vi "FLS.vi"(0 "System no.":i32=1 min=1 step=1, 1 "Board":i32=1 min=1 max=5 step=1, 2 "Axis to scan":string, 3 "Scan direction":u16(ring)=2 items=["Scan left & right (- & +)", "Scan only left (-)", "Scan only right (+)"], 4 "Range":dbl=0.1 format="%.4f", 5 "error in":errorcluster, 6 "Treshold level":dbl=0.1 format="%.3f", 7 "Step size":dbl=0.001 format="%.4f", 8 "Decrease VEL\nfor scan?":bool, 9 "Velocity":dbl=0.2 format="%.4f", 10 "Use #7 polling?":bool=TRUE, 11 "Timeout (s)":dbl=300.0 min=1.0 max=4.0 step=1.0 format="%.2f", 12 "Stop refnum":refnum<vi>) -> (14 "Scan successful?":bool, 15 "Controller error":bool, 19 "error out":errorcluster)   [LabVIEW 2026]
doc: "Performs a line scan specified axis, waits until scan is ready (using #7 polling if checked) and indicates whether scan was successful or not. Velocity is only valid if Decrease VEL for scan? Is TRUE. If Decrease VEL for scan? is TRUE, velocity is decreased before and reset after the scan. Timeout is only valid if Use #7 polling is FALSE. If Refnum stop or Local stop is TRUE, VI sends #24 and stops. When using as a sub-VI, use Refnum stop to stop VI from caller.\n\nC-880: Use #7 polling? = TRUE\n\nC-887, F-206, M-8X0: Use #7 polling? = FALSE. Only for GCS syntax version = GCS 2.0 or higher (check with CSV?.vi. If CSV?.vi is not supported, syntax version is GCS 1.0). Step size is not valid."
uses:
  Communication/Syntax.ctl
  GeneralCommands/Controller names.ctl
  Communication/Global1.vi
  GeneralCommands/Global2 (Array).vi
panel:
  in  "Local stop":bool
  # "Performs a line scan in specified axis, waits until scan is ready (using #7 polling if \nchecked) and indicates whether scan was successful or not. If Stop refnum or \nLocal stop is TRUE, VI sends #24 and stops. \"Velocity\" is only valid if \"Decrease VEL \nfor scan?\" Is TRUE.  If \"Decrease VEL for scan?\" is TRUE, velocity is decreased before \nand reset after the scan. \"Timeout\" is only valid if \"Use #7 polling\" is FALSE."
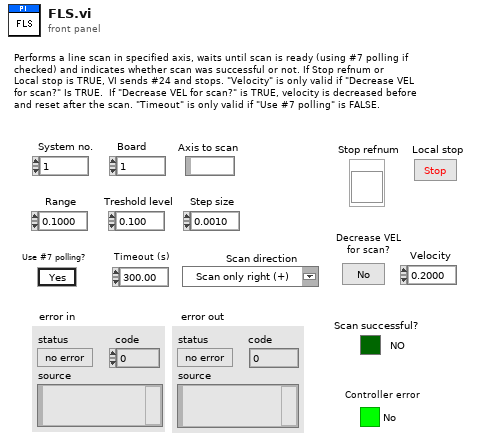
[diagram p1: front panel]
types:
  T1 = typedef "Syntax.ctl" = enum16{"GCS 1.0", "GCS 2.0", "GCS 3.0"}
  T2 = typedef "Controller names.ctl" = enum16{"None", "Analog", "C-702", "C-413", "C-414", "C-843", "C-843.PM", "C-844", "C-848", "C-865", "C-866", "C-867", "C-877", "C-880", "C-884", "C-885", "C-886", "C-887", "C-891", "E-135", "E-516", "E-517", "E-518", "E-709", "E-710", "E-712", "E-725", "E-727", "E-753", "E-754", "E-755", "E-761", "E-816", "E-861", "E-870", "E-871", "E-872", "E-873", "E-874", "F-206", "HydraPollux", "M-840", "M-850", "M-8X0", "Mercury", "Mercury_GCS", "PI_GCS2"}
  T3 = cluster{"Conn. axes":string[], "Controller name":T2}[]
  T4 = cluster{"Conn. axes":string[], "Controller name":T2}
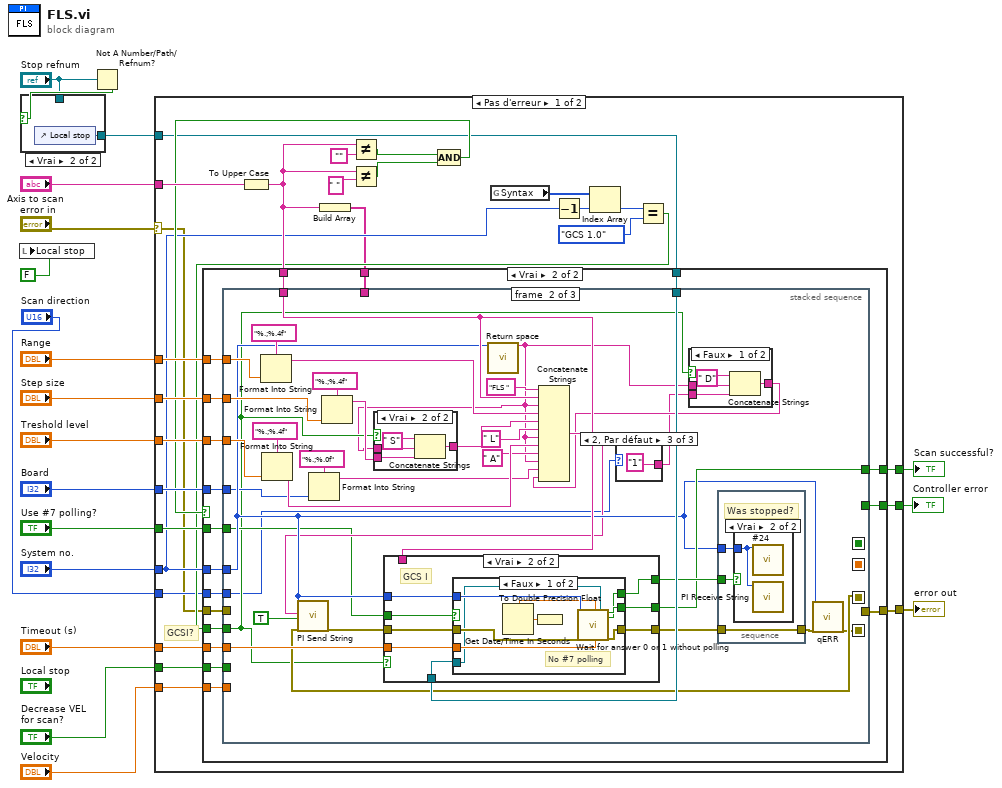
[diagram p0: block diagram]
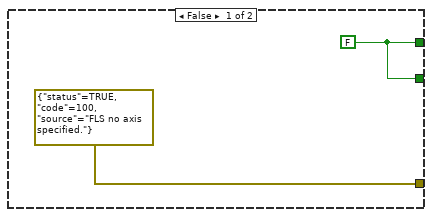
[diagram p3: hidden frame]
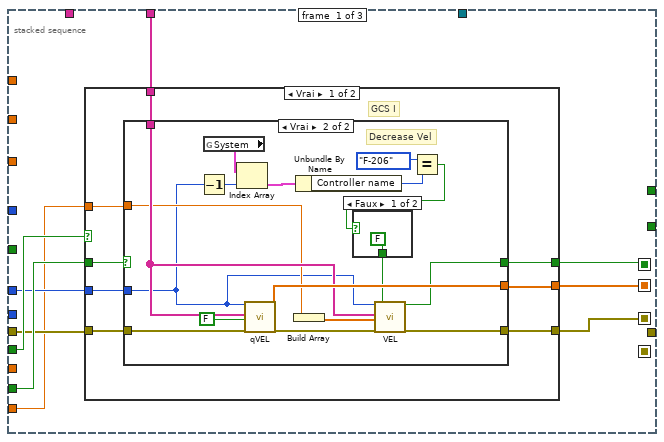
[diagram p4: hidden frame]
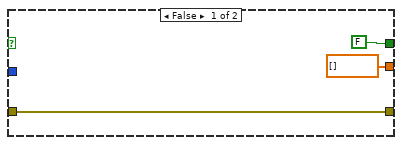
[diagram p5: hidden frame]
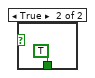
[diagram p6: hidden frame]
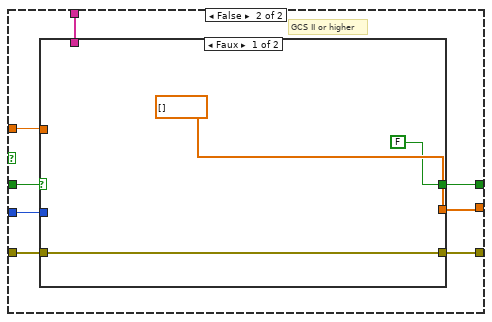
[diagram p7: hidden frame]
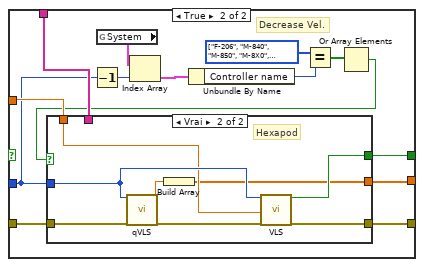
[diagram p8: hidden frame]
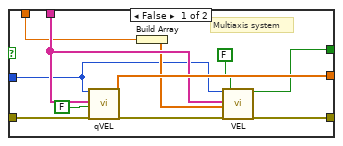
[diagram p9: hidden frame]
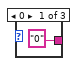
[diagram p10: hidden frame]
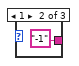
[diagram p11: hidden frame]
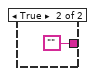
[diagram p12: hidden frame]
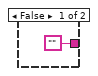
[diagram p13: hidden frame]
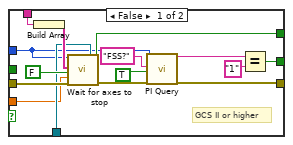
[diagram p14: hidden frame]
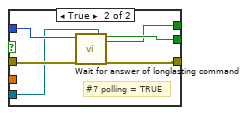
[diagram p15: hidden frame]
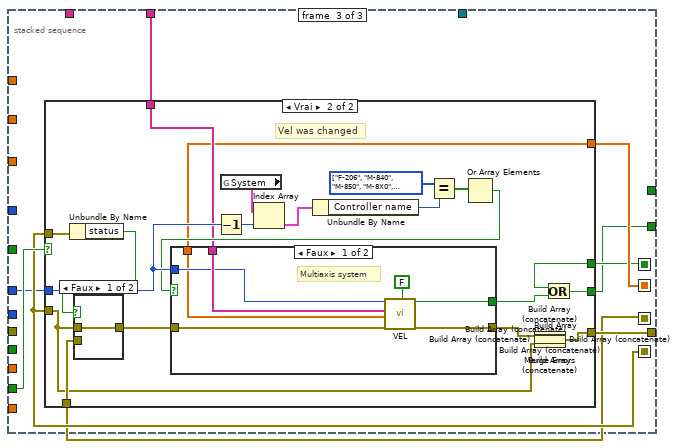
[diagram p17: hidden frame]
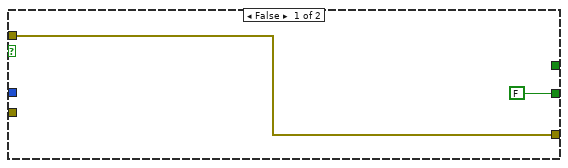
[diagram p18: hidden frame]
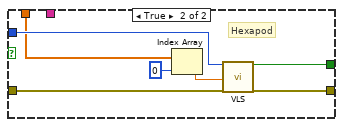
[diagram p19: hidden frame]
diagram:
  n1 = local write "Local stop"(FALSE ("Local stop")) -> ()
  n2 = Not A Number/Path/Refnum?(number/path/refnum="Stop refnum") -> (NaN/Path/Refnum?=w10:bool)
  n3 = case shown="Vrai" w10 {
    tunnel: [w20 w21] -> w8
    tunnel: "Stop refnum" -> [w20 _]
    frame False {
    }
    frame True {
      n4 = control-ref of="Local stop"() -> (w21:refnum<vi>)
    }
  }
  n5 = case shown="Pas d'erreur" "error in" {
    selector: "error in" -> [w23 w297]
    tunnel: "System no." -> [w30 _]
    tunnel: [w38 w297] -> w18
    tunnel: "Axis to scan" -> [w49 _]
    tunnel: [w37 w298] -> w16
    tunnel: "Board" -> [w44 _]
    tunnel: "Range" -> [w43 _]
    tunnel: "Step size" -> [w42 _]
    tunnel: "Treshold level" -> [w40 _]
    tunnel: w8 -> [w36 _]
    tunnel: "Use #7 polling?" -> [w35 _]
    tunnel: "Timeout (s)" -> [w34 _]
    tunnel: "Decrease VEL\nfor scan?" -> [w28 _]
    tunnel: "Velocity" -> [w27 _]
    tunnel: [w25 w298] -> w3
    tunnel: "Scan direction" -> [w24 _]
    frame No Error {
      # "GCSI?"
      n6 = To Upper Case(1:w49) -> (0:w41:string)
      n7 = Build Array(w41) -> (w26:string[])
      n8 = Not Equal?(x=w41, y="") -> (x != y?=w46:bool)
      n9 = Not Equal?(x=w41, y=" ") -> (x != y?=w45:bool)
      n10 = Compound Arithmetic op=AND(w46, w45) -> (w39:bool)
      n11 = global read "Global1.vi" "Syntax"() -> (w31:T1[])
      n12 = Decrement(x=w30) -> (x-1=w32:i32)
      n13 = Index Array(array=w31, index=w32) -> (element=w33:T1)
      n14 = Equal?(x=w33, y=Syntax."GCS 1.0") -> (x = y?=w29:bool)
      n15 = case shown="Vrai" w39 {
        tunnel: w44 -> [_ w58]
        tunnel: w43 -> [_ w68]
        tunnel: w42 -> [_ w66]
        tunnel: w41 -> [_ w63]
        tunnel: w40 -> [_ w67]
        tunnel: w23 -> [_ w69]
        tunnel: w30 -> [_ w59]
        tunnel: [errorcluster {"status"=TRUE, "code"=100, "source"="FLS no axis specified."} ("error out") w65] -> w38
        tunnel: [w50 w61] -> w37
        tunnel: w36 -> [_ w62]
        tunnel: w35 -> [_ w64]
        tunnel: w34 -> [_ w60]
        tunnel: w29 -> [_ w57]
        tunnel: w28 -> [_ w56]
        tunnel: w27 -> [_ w55]
        tunnel: w26 -> [_ w54]
        tunnel: [w50 w53] -> w25
        tunnel: w24 -> [_ w52]
        frame False {
          w50 = FALSE
        }
        frame True {
          n16 = stacked-sequence {
            seq-local: [w74 _ _] -> [_ w162 w247]
            seq-local: [w73 _ _] -> [_ _ w244]
            seq-local: [w70 _ _] -> [_ _ w245]
            seq-local: [_ w161 _] -> [_ _ w249]
            tunnel: w69 -> [w75 _ _]
            tunnel: w68 -> [_ w185 _]
            tunnel: w67 -> [_ w182 _]
            tunnel: w66 -> [_ w180 _]
            tunnel: [_ _ w250] -> w65
            tunnel: w64 -> [_ w160 _]
            tunnel: w63 -> [_ w174 _]
            tunnel: w62 -> [_ w173 _]
            tunnel: [_ w170 _] -> w61
            tunnel: w60 -> [_ w169 _]
            tunnel: w59 -> [w76 w168 w248]
            tunnel: w58 -> [_ w165 _]
            tunnel: w57 -> [w78 w156 _]
            tunnel: w56 -> [w77 _ w251]
            tunnel: w55 -> [w72 _ _]
            tunnel: w54 -> [w71 _ w246]
            tunnel: [_ _ w243] -> w53
            tunnel: w52 -> [_ w154 _]
            frame #0 {
              n17 = case shown="Vrai" w78 {
                tunnel: w71 -> [w83 w113]
                tunnel: w75 -> [w86 w116]
                tunnel: [w85 w115] -> w70
                tunnel: w76 -> [w80 w110]
                tunnel: [w84 w114] -> w74
                tunnel: w72 -> [w82 w112]
                tunnel: [w81 w111] -> w73
                tunnel: w77 -> [w79 w109]
                frame True {
                  # "GCS I"
                  n18 = case shown="Vrai" w79 {
                    tunnel: w86 -> [w87 w105]
                    tunnel: [dbl[] [] ("Velocity") w104] -> w85
                    tunnel: [w87 w102] -> w84
                    tunnel: w83 -> [_ w101]
                    tunnel: w82 -> [_ w100]
                    tunnel: [FALSE ("Controller error") w98] -> w81
                    tunnel: w80 -> [_ w96]
                    frame False {
                    }
                    frame True {
                      # "Decrease Vel"
                      n19 = Decrement(x=w96) -> (x-1=w95:i32)
                      n20 = global read "Global2 (Array).vi" "System"() -> (w97:T3)
                      n21 = Index Array(array=w97, index=w95) -> (element=w94:T4)
                      n22 = call "qVEL.vi"("System no."=w96, "Axes to query"=w101, "All axes?"=FALSE, "error in"=w105) -> ("Velocity"=w104:dbl[], "error out"=w103:errorcluster)  [unwired: 1 in, 13 out]
                      n23 = Build Array(w100) -> (w99:dbl[])
                      n24 = Unbundle By Name(w94) -> ("Controller name"=w93:T2)
                      n25 = Equal?(x=Controller_names."F-206" ("Controller name"), y=w93) -> (x = y?=w91:bool)
                      n26 = case shown="Faux" w91 {
                        tunnel: [FALSE ("Without axis ID?") TRUE ("Without axis ID?")] -> w90
                        frame False {
                        }
                        frame True {
                        }
                      }
                      n27 = call "VEL.vi"("System no."=w96, "Axes to set"=w101, "Velocity values"=w99, "error in"=w103, "Without axis ID?"=w90) -> ("Controller error"=w98:bool, "error out"=w102:errorcluster)  [unwired: 1 in, 12 out]
                    }
                  }
                }
                frame False {
                  # "GCS II or higher"
                  n28 = case shown="Faux" w109 {
                    tunnel: w116 -> [w117 w133]
                    tunnel: [dbl[] [] ("Velocity") w132] -> w115
                    tunnel: [w117 w131] -> w114
                    tunnel: w113 -> [_ w130]
                    tunnel: w112 -> [_ w129]
                    tunnel: [FALSE ("Controller error") w128] -> w111
                    tunnel: w110 -> [_ w126]
                    frame False {
                    }
                    frame True {
                      w122 = T2[] [enum."F-206", enum."M-840", enum."M-850", enum."M-8X0", enum."C-887"] items=["None", "Analog", "C-702", "C-413", "C-414", "C-843", "C-843.PM", "C-844", "C-848", "C-865", "C-866", "C-867", "C-877", "C-880", "C-884", "C-885", "C-886", "C-887", "C-891", "E-135", "E-516", "E-517", "E-518", "E-709", "E-710", "E-712", "E-725", "E-727", "E-753", "E-754", "E-755", "E-761", "E-816", "E-861", "E-870", "E-871", "E-872", "E-873", "E-874", "F-206", "HydraPollux", "M-840", "M-850", "M-8X0", "Mercury", "Mercury_GCS", "PI_GCS2"]
                      # "Decrease Vel."
                      n29 = Decrement(x=w126) -> (x-1=w125:i32)
                      n30 = global read "Global2 (Array).vi" "System"() -> (w127:T3)
                      n31 = Index Array(array=w127, index=w125) -> (element=w124:T4)
                      n32 = Unbundle By Name(w124) -> ("Controller name"=w123:T2)
                      n33 = Equal?(x=w122, y=w123) -> (x = y?=w121:bool[])
                      n34 = Or Array Elements(Boolean array=w121) -> (logical OR=w120:bool)
                      n35 = case shown="Vrai" w120 {
                        tunnel: w133 -> [w143 w152]
                        tunnel: [w142 w145] -> w132
                        tunnel: [w140 w150] -> w131
                        tunnel: w130 -> [w139 _]
                        tunnel: w129 -> [w138 w147]
                        tunnel: [w136 w149] -> w128
                        tunnel: w126 -> [w135 w148]
                        frame False {
                          # "Multiaxis system"
                          n36 = call "qVEL.vi"("System no."=w135, "Axes to query"=w139, "All axes?"=FALSE, "error in"=w143) -> ("Velocity"=w142:dbl[], "error out"=w141:errorcluster)  [unwired: 1 in, 13 out]
                          n37 = Build Array(w138) -> (w137:dbl[])
                          n38 = call "VEL.vi"("System no."=w135, "Axes to set"=w139, "Velocity values"=w137, "error in"=w141, "Without axis ID?"=FALSE) -> ("Controller error"=w136:bool, "error out"=w140:errorcluster)  [unwired: 1 in, 12 out]
                        }
                        frame True {
                          # "Hexapod"
                          n39 = call "qVLS.vi"("System no."=w148, "error in"=w152) -> ("Velocity"=w146:dbl, "error out"=w151:errorcluster)  [unwired: 2 in, 14 out]
                          n40 = Build Array(w146) -> (w145:dbl[])
                          n41 = call "VLS.vi"("System no."=w148, "Velocity"=w147, "error in"=w151) -> ("Controller error"=w149:bool, "error out"=w150:errorcluster)  [unwired: 3 in, 12 out]
                        }
                      }
                    }
                  }
                }
              }
            }
            frame #1 {
              n42 = Format Into String(format string="%.;%.4f" ("Format String"), w185) -> (resulting string=w184:string)  [unwired: 2 in, 1 out]
              n43 = Format Into String(format string="%.;%.4f" ("Format String"), w182) -> (resulting string=w179:string)  [unwired: 2 in, 1 out]
              n44 = Format Into String(format string="%.;%.0f" ("Format String"), w165) -> (resulting string=w164:string)  [unwired: 2 in, 1 out]
              n45 = Format Into String(format string="%.;%.4f" ("Format String"), w180) -> (resulting string=w159:string)  [unwired: 2 in, 1 out]
              n46 = call "Return space.vi"("System no."=w168) -> ("String out"=w155:string)  [unwired: 1 in, 17 out]
              n47 = case shown="Vrai" w156 {
                tunnel: ["" w200] -> w158
                tunnel: w155 -> [_ w198]
                tunnel: w159 -> [_ w197]
                frame False {
                }
                frame True {
                  n48 = Concatenate Strings(" S", w198, w197) -> (w200:string)
                }
              }
              n49 = case shown="2, Par défaut" w154 {
                tunnel: ["0" "-1" "1"] -> w153
                frame 0 {
                }
                frame 1 {
                }
                frame 2, Default {
                }
              }
              n50 = case shown="Faux" w156 {
                tunnel: [w194 ""] -> w157
                tunnel: w155 -> [w192 _]
                tunnel: w153 -> [w191 _]
                frame False {
                  n51 = Concatenate Strings(" D", w192, w191) -> (w194:string)
                }
                frame True {
                }
              }
              n52 = Concatenate Strings("FLS ", w174, w155, w184, w158, " L", w155, w179, " A" ("Substring"), w155, w164, w157) -> (w163:string)
              n53 = call "PI Send String.vi"("System no."=w168, "String to send"=w163, "Attach termination char.?"=TRUE ("Attach Linefeed?"), "error in"=w162) -> ("error out"=w175:errorcluster)  [unwired: 15 out]
              n54 = case shown="Vrai" w156 {
                tunnel: w160 -> [_ w223]
                tunnel: w169 -> [w203 w222]
                tunnel: [w201 w221] -> w172
                tunnel: [w204 w220] -> w170
                tunnel: w173 -> [w211 w219]
                tunnel: [w210 w218] -> w171
                tunnel: w168 -> [w206 w217]
                tunnel: w175 -> [w214 w216]
                tunnel: w174 -> [w212 _]
                frame False {
                  # "GCS II or higher"
                  n55 = Build Array(w212) -> (w213:string[])
                  n56 = call "Wait for axes to stop.vi"("System no."=w206, "Axes to wait for"=w213, "With status bit polling?"=FALSE, "Timeout (s)"=w203, "error in"=w214, "Stop refnum"=w211) -> ("Stopped"=w210:bool, "error out"=w207:errorcluster)  [unwired: 1 in, 11 out]
                  n57 = call "PI Query.vi"("System no."=w206, "String to send"="FSS?", "Attach termination char.?"=TRUE ("Attach Linefeed?"), "error in"=w207) -> ("String read"=w202:string, "error out"=w201:errorcluster)  [unwired: 3 in, 11 out]
                  n58 = Equal?(x=w202, y="1") -> (x = y?=w204:bool)
                }
                frame True {
                  # "GCS I"
                  n59 = case shown="Faux" w223 {
                    tunnel: w217 -> [w232 w238]
                    tunnel: w216 -> [w231 w237]
                    tunnel: [w230 w236] -> w221
                    tunnel: [w229 w235] -> w220
                    tunnel: w222 -> [w227 _]
                    tunnel: w219 -> [w226 w234]
                    tunnel: [w225 w233] -> w218
                    frame False {
                      # "No #7 polling"
                      n60 = Get Date/Time In Seconds() -> (seconds since 1Jan1904=w224:timestamp)
                      n61 = To Double Precision Float(number=w224) -> (double precision float=w228:dbl)
                      n62 = call "Wait for answer 0 or 1 without polling.vi"("System no."=w232, "error in"=w231, "Start time"=w228, "Timeout (s)"=w227, "Stop refnum"=w226) -> ("Scan successful?"=w229:bool, "Stopped"=w225:bool, "error out"=w230:errorcluster)  [unwired: 12 out]
                    }
                    frame True {
                      # "#7 polling = TRUE"
                      n63 = call "Wait for answer of longlasting command.vi"("System no."=w238, "error in"=w237, "Stop refnum"=w234) -> ("Answer"=w235:bool, "Stopped"=w233:bool, "error out"=w236:errorcluster)  [unwired: 14 out]
                    }
                  }
                }
              }
              n64 = stacked-sequence {
                tunnel: w168 -> [w241]
                tunnel: [w240] -> w177
                tunnel: w172 -> [w240]
                tunnel: w171 -> [w239]
                frame #0 {
                  # "Was stopped?"
                  n65 = case shown="Vrai" w239 {
                    tunnel: w241 -> [_ w242]
                    frame False {
                    }
                    frame True {
                      n66 = call "#24.vi"("System no."=w242) -> ()  [unwired: 1 in, 18 out]
                      n67 = call "PI Receive String.vi"("System no."=w242) -> ()  [unwired: 2 in, 17 out]
                    }
                  }
                }
              }
              n68 = call "qERR.vi"("System no."=w168, "error in"=w177) -> ("error out"=w161:errorcluster)  [unwired: 17 out]
            }
            frame #2 {
              n69 = case shown="Vrai" w251 {
                tunnel: w249 -> [w253 w280]
                tunnel: [w253 w262] -> w250
                tunnel: w249 -> [_ w261]
                tunnel: w248 -> [_ w279]
                tunnel: w247 -> [_ w278]
                tunnel: w246 -> [_ w270]
                tunnel: w245 -> [_ w269]
                tunnel: w244 -> [_ w266]
                tunnel: [FALSE w265] -> w243
                frame False {
                }
                frame True {
                  w273 = T2[] [enum."F-206", enum."M-840", enum."M-850", enum."M-8X0", enum."C-887"] items=["None", "Analog", "C-702", "C-413", "C-414", "C-843", "C-843.PM", "C-844", "C-848", "C-865", "C-866", "C-867", "C-877", "C-880", "C-884", "C-885", "C-886", "C-887", "C-891", "E-135", "E-516", "E-517", "E-518", "E-709", "E-710", "E-712", "E-725", "E-727", "E-753", "E-754", "E-755", "E-761", "E-816", "E-861", "E-870", "E-871", "E-872", "E-873", "E-874", "F-206", "HydraPollux", "M-840", "M-850", "M-8X0", "Mercury", "Mercury_GCS", "PI_GCS2"]
                  # "Vel was changed"
                  n70 = Unbundle By Name(w280) -> ("status"=w264:bool)
                  n71 = case shown="Faux" w264 {
                    tunnel: w261 -> [w295 _]
                    tunnel: [w295 w296] -> w268
                    tunnel: w278 -> [_ w296]
                    frame False {
                    }
                    frame True {
                    }
                  }
                  n72 = Decrement(x=w279) -> (x-1=w276:i32)
                  n73 = global read "Global2 (Array).vi" "System"() -> (w277:T3)
                  n74 = Index Array(array=w277, index=w276) -> (element=w275:T4)
                  n75 = Unbundle By Name(w275) -> ("Controller name"=w274:T2)
                  n76 = Equal?(x=w273, y=w274) -> (x = y?=w272:bool[])
                  n77 = Or Array Elements(Boolean array=w272) -> (logical OR=w271:bool)
                  n78 = case shown="Faux" w271 {
                    tunnel: w268 -> [w282 w292]
                    tunnel: [w287 w288] -> w263
                    tunnel: w270 -> [w286 _]
                    tunnel: w269 -> [w281 w290]
                    tunnel: [w285 w294] -> w267
                    tunnel: w279 -> [w284 w293]
                    frame False {
                      # "Multiaxis system"
                      n79 = call "VEL.vi"("System no."=w284, "Axes to set"=w286, "Velocity values"=w281, "error in"=w282, "Without axis ID?"=FALSE) -> ("Controller error"=w285:bool, "error out"=w287:errorcluster)  [unwired: 1 in, 12 out]
                    }
                    frame True {
                      # "Hexapod"
                      n80 = Index Array(array=w290, index=0) -> (element=w291:dbl)
                      n81 = call "VLS.vi"("System no."=w293, "Velocity"=w291, "error in"=w292) -> ("Controller error"=w294:bool, "error out"=w288:errorcluster)  [unwired: 3 in, 12 out]
                    }
                  }
                  n82 = Build Array(w263, w261) -> (w260:errorcluster[])
                  n83 = Build Array (concatenate)(w260) -> (w259:errorcluster[])
                  n84 = Build Array (concatenate)(w259) -> (w258:errorcluster[])
                  n85 = Build Array (concatenate)(w258) -> (w257:errorcluster[])
                  n86 = Build Array (concatenate)(w257) -> (w256:errorcluster[])
                  n87 = Build Array (concatenate)(w256) -> (w255:errorcluster[])
                  n88 = Build Array (concatenate)(w255) -> (w254:errorcluster[])
                  n89 = Merge Errors(w254) -> (w262:errorcluster)
                  n90 = Or(x=w266, y=w267) -> (x .or. y?=w265:bool)
                }
              }
            }
          }
        }
      }
    }
    frame Error {
      w298 = FALSE
    }
  }
  "error out" <- w18
  "Scan successful?" <- w16
  "Controller error" <- w3
